vi "Queue Driver.vi"(0 "Name":string, 5 "State In N":string[](array[string]), 7 "State In":string, 11 "Error In":errorcluster, 13 "Enum":T1) -> (4 "State Out":string, 15 "Error Out":errorcluster)   [LabVIEW 2020, in "String based State machine - Airplane.lvlib"]
doc: "This VI is a LV2, which is used to create Queue driver."
uses:
  String based State machine - Airplane.lvlib
  Queue Drive mode.ctl
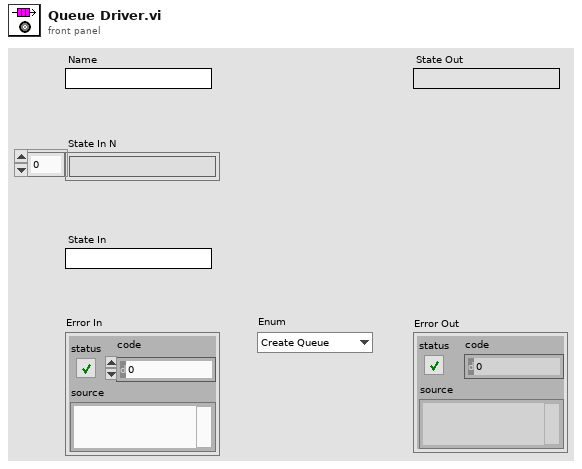
[diagram p1: front panel]
types:
  T1 = typedef "String based State machine - Airplane.lvlib/Queue Drive mode.ctl" = enum16{"Create Queue", "Release Queue", "Enqueue N", "Flush Queue", "Enstack", "Dequeue", "Enqueue"}
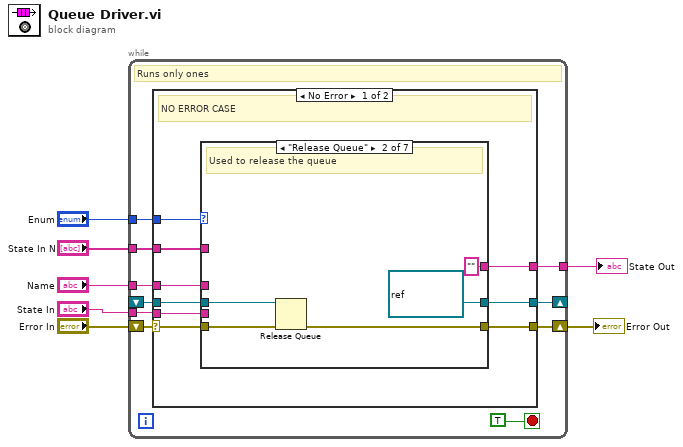
[diagram p0: block diagram]
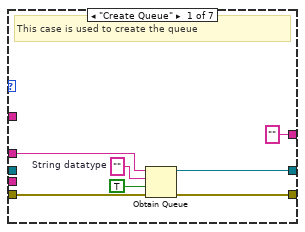
[diagram p2: hidden frame]
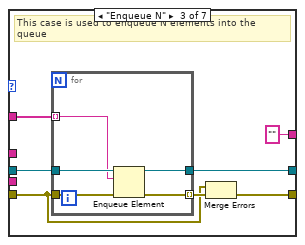
[diagram p3: hidden frame]
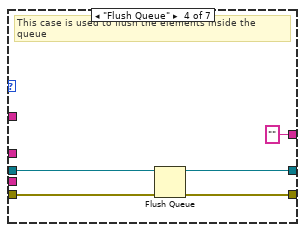
[diagram p4: hidden frame]
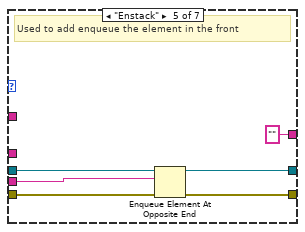
[diagram p5: hidden frame]
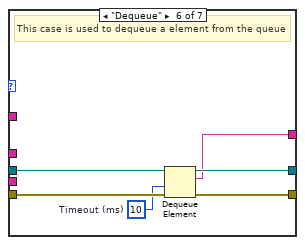
[diagram p6: hidden frame]
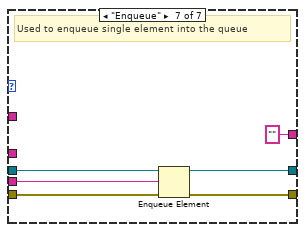
[diagram p7: hidden frame]
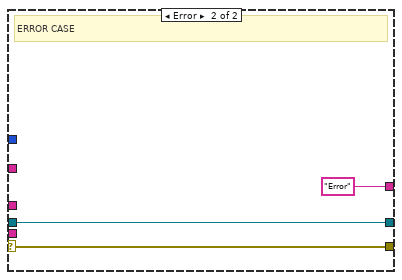
[diagram p8: hidden frame]
diagram:
  n1 = while {
    tunnel: "Enum" -> [w15]
    tunnel: "State In" -> [w13]
    tunnel: "State In N" -> [w12]
    shift-right: [w16] -> w6
    shift-left: "Error In" -> [w17]
    tunnel: "Name" -> [w14]
    tunnel: [w11] -> w1
    shift-right: [w9] -> _
    shift-left: _ -> [w10]
    stop <- TRUE stop-if-true
    # "Runs only ones"
    n2 = case shown="No Error" w17 {
      selector: w17 -> [w25 w76]
      tunnel: [w26 w76] -> w16
      tunnel: w15 -> [w24 _]
      tunnel: w14 -> [w23 _]
      tunnel: w13 -> [w22 _]
      tunnel: w12 -> [w21 _]
      tunnel: [w20 "Error"] -> w11
      tunnel: w10 -> [w19 w74]
      tunnel: [w18 w74] -> w9
      frame No Error {
        # "NO ERROR CASE"
        n3 = case shown="\"Release Queue\"" w24 {
          tunnel: [w33 w38 w40 w55 w61 w67 w73] -> w26
          tunnel: w25 -> [w32 w37 w39 w54 w60 w66 w72]
          tunnel: w23 -> [w31 _ _ _ _ _ _]
          tunnel: [w28 refnum<queue> refnum ("queue out") w43 w52 w57 w64 w69] -> w18
          tunnel: w19 -> [_ w36 w44 w53 w59 w65 w70]
          tunnel: w22 -> [_ _ _ _ w58 _ w71]
          tunnel: w21 -> [_ _ w42 _ _ _ _]
          tunnel: ["" "" "" "" "" w63 ""] -> w20
          frame "Create Queue" {
            w29 = ""  # String datatype
            # "This case is used to create the queue"
            n4 = Obtain Queue(name (unnamed)=w31, element data type=w29, create if not found? (T)=TRUE, error in (no error)=w32) -> (queue out=w28:refnum<queue>, error out=w33:errorcluster)  [unwired: 1 in, 1 out]
          }
          frame "Release Queue" {
            # "Used to release the queue"
            n5 = Release Queue(queue=w36, error in (no error)=w37) -> (error out=w38:errorcluster)  [unwired: 1 in, 2 out]
          }
          frame "Enqueue N" {
            # "This case is used to enqueue N elements into the queue"
            n6 = for {
              tunnel: w44 -> [w48]
              tunnel: [w47] -> w43
              tunnel: w42 -> [w46] mode=indexing
              tunnel: w39 -> [w49]
              tunnel: [w50] -> w45 mode=indexing
              n7 = Enqueue Element(queue=w48, element=w46, error in (no error)=w49) -> (queue out=w47:refnum<queue>, error out=w50:errorcluster)  [unwired: 1 in, 1 out]
            }
            n8 = Merge Errors(w39, w45) -> (w40:errorcluster)
          }
          frame "Flush Queue" {
            # "This case is used to flush the elements inside the queue"
            n9 = Flush Queue(queue=w53, error in (no error)=w54) -> (queue out=w52:refnum<queue>, error out=w55:errorcluster)  [unwired: 1 out]
          }
          frame "Enstack" {
            # "Used to add enqueue the element in the front"
            n10 = Enqueue Element At Opposite End(queue=w59, element=w58, error in (no error)=w60) -> (queue out=w57:refnum<queue>, error out=w61:errorcluster)  [unwired: 1 in, 1 out]
          }
          frame "Dequeue" {
            w62 = 10  # Timeout (ms)
            # "This case is used to dequeue a element from the queue"
            n11 = Dequeue Element(queue=w65, timeout in ms (-1)=w62, error in (no error)=w66) -> (queue out=w64:refnum<queue>, element=w63:string, error out=w67:errorcluster)  [unwired: 1 out]
          }
          frame "Enqueue" {
            # "Used to enqueue single element into the queue"
            n12 = Enqueue Element(queue=w70, element=w71, error in (no error)=w72) -> (queue out=w69:refnum<queue>, error out=w73:errorcluster)  [unwired: 1 in, 1 out]
          }
        }
      }
      frame Error {
        # "ERROR CASE"
      }
    }
  }
  "Error Out" <- w6
  "State Out" <- w1
